vi "Data Processor.vi"() -> (0 "Data Export":T5 {"Data Channels" format="%.2f"})   [LabVIEW 2016]
uses:
  state.ctl
  comm/comm.lvlib
panel:
  in  "LE and RE 2D coils":bool
  in  "Case Constant\n(See Context Help)":bool=TRUE
  in  "3D Convention":T1(ring)=enum."Rotation Vectors"
  in  "Sub Sample Once":bool
  in  "Rex Data File":T2 {"Data -> Additional" format="%.2f"; "Data -> 3D Coil" format="%.2f"}
  in  "Addtional Channels":T3(array[cluster])=[{"Channel No."=0, "Offset Factor"=0.0, "Scaling Factor"=1.0}, {"Channel No."=19, "Offset Factor"=0.0, "Scaling Factor"=1.0}, {"Channel No."=20, "Offset Factor"=0.0, "Scaling Factor"=1.0}, {"Channel No."=21, "Offset Factor"=0.0, "Scaling Factor"=0.1}, {"Channel No."=22, "Offset Factor"=0.0, "Scaling Factor"=0.1}, {"Channel No."=23, "Offset Factor"=0.0, "Scaling Factor"=0.1}, {"Channel No."=24, "Offset Factor"=0.0, "Scaling Factor"=3.05e-05}, {"Channel No."=25, "Offset Factor"=0.0, "Scaling Factor"=3.05e-05}, {"Channel No."=26, "Offset Factor"=0.0, "Scaling Factor"=3.05e-05}, {"Channel No."=27, "Offset Factor"=0.0, "Scaling Factor"=3.05e-05}, {"Channel No."=28, "Offset Factor"=0.0, "Scaling Factor"=1.0}] {"Scaling Factor" format="%.7f"; "Offset Factor" format="%.2f"}
  in  "Coil 0 (Head) : Coil 1 (Left Eye) : Coil 2 (Right Eye)":T4(array[cluster])=[{"Dir and X field channel No."=9, "Dir and Y field channel No."=7, "Dir and Z field channel No."=8, "Tor and X field channel No."=18, "Tor and Y field channel No."=16, "Tor and Z field channel No."=17, "Common Offset Factor"=2048.0, "Common Scaling Factor"=1.0}, {"Dir and X field channel No."=12, "Dir and Y field channel No."=10, "Dir and Z field channel No."=11, "Tor and X field channel No."=15, "Tor and Y field channel No."=13, "Tor and Z field channel No."=14, "Common Offset Factor"=2048.0, "Common Scaling Factor"=1.0}, {"Dir and X field channel No."=3, "Dir and Y field channel No."=1, "Dir and Z field channel No."=2, "Tor and X field channel No."=6, "Tor and Y field channel No."=4, "Tor and Z field channel No."=5, "Common Offset Factor"=2048.0, "Common Scaling Factor"=1.0}] {"Common Scaling Factor" format="%.2f"; "Common Offset Factor" format="%.2f"}
  in  "Export Channel List":u16[](array[ring])=[0, 1, 2, 9, 10, 11, 12, 13, 3, 4, 5, 14, 15, 16, 17, 18, 6, 7, 8, 19, 20, 21, 22, 23, 26, 27, 28, 29, 30, 31, 34, 24, 25, 38] items=["Hz Position-in-Head", "Hy Position-in-Head", "Hx Position-in-Head", "Lz Position-in-Head", "Ly Position-in-Head", "Lx Position-in-Head", "Rz Position-in-Head", "Ry Position-in-Head", "Rx Position-in-Head", "Hx Velocity-in-Head", "Hy Velocity-in-Head", "Hz Velocity-in-Head", "Hl Velocity-in-Head", "Hr Velocity-in-Head", "Lx Velocity-in-Head", "Ly Velocity-in-Head", "Lz Velocity-in-Head", "Ll Velocity-in-Head", "Lr Velocity-in-Head", "Rx Velocity-in-Head", "Ry Velocity-in-Head", "Rz Velocity-in-Head", "Rl Velocity-in-Head", "Rr Velocity-in-Head", "Chair Position", "Chair Velocity", "Button", "Ascension X or ch25", "Ascension X Vel", "Ascension Y", "Ascension Y Vel", "Ascension Z", "Ascension Z Vel", "Ascension q0", "Ascension q1", "Ascension q2", "Ascension q3", "LED", " "]
  out "Processing":bool
  out "All Data":T5 {"Data Channels" format="%.2f"}
  in  "Manually enter the Field Gains":bool
  in  "Selected Calibration File":string
  in  "Calibration File":bool
  in  "Field Gains":i32[][](array[numeric])
  in  "Start Processing":bool
  in  "Channel Plot DY DZ for H LE RE":i32[](array[numeric])=[1, 2, 7, 8, 13, 14, 20]
  in  "Selected Data File":string
  in  "Data File":bool
  in  "Quit":bool
  in  "Stop":bool
  # "Human Data Processor"
  # "AAM 10 april 2002 ver.10"
  # "Coil 2                                   Coil 1                                  Coil 0\n              D                  T                     D                  T                   D                    T"
  # "X"
  # "Y"
  # "Z"
  # "NOTE: EMPTY LIST ALWAYS AT END"
  # "Copyright Americo A. Migliaccio (c) 2002 All Rights Reserved by Author"
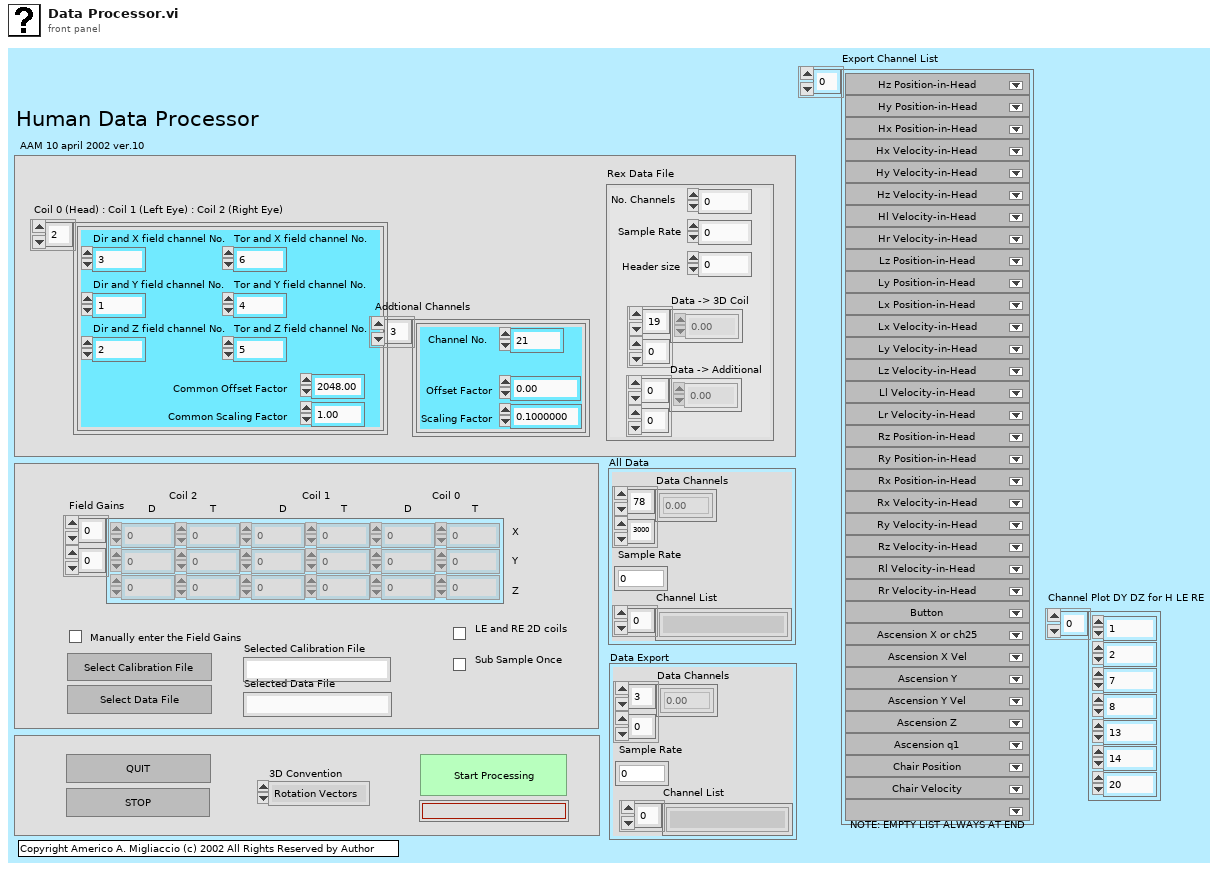
[diagram p1: front panel]
types:
  T1 = enum16{"Rotation Matrix", "Rotation Vectors", "Quaternions", "Fick Angles", "Helmholtz Angles"}
  T2 = cluster{"Header size":i32, "No. Channels":i32, "Sample Rate":i32, "Data -> 3D Coil":dbl[][], "Data -> Additional":dbl[][]}
  T3 = cluster{"Channel No.":i32, "Offset Factor":dbl, "Scaling Factor":dbl}[]
  T4 = cluster{"Dir and X field channel No.":i32, "Dir and Y field channel No.":i32, "Dir and Z field channel No.":i32, "Tor and X field channel No.":i32, "Tor and Y field channel No.":i32, "Tor and Z field channel No.":i32, "Common Offset Factor":dbl, "Common Scaling Factor":dbl}[]
  T5 = cluster{"Data Channels":dbl[][], "Sample Rate":i32, "Channel List":string[]}
  T6 = typedef "state.ctl" = enum16{"Calculate 6 Field/Int Rot Matrix", "SubSample", "Panel Monitoring", "Initialize", "Read 6 Field/Int Calibration File", "Read 6 Field/Int Data File", "Sort 6 Field/Int Channels", "Export Channels", "Stop", "Quit"}
  T7 = enum16{"Position in Space", "Position in Head", "Position in Eye", "Velocity in Space", "Velocity in Head", "Velocity in Eye", "Acceleration in Space", "Acceleration in Head"}
  T8 = cluster{"Coil 0 (Head) : Coil 1 (Left Eye) : Coil 2 (Right Eye)":cluster{"Dir and X field channel No.":i32, "Dir and Y field channel No.":i32, "Dir and Z field channel No.":i32, "Tor and X field channel No.":i32, "Tor and Y field channel No.":i32, "Tor and Z field channel No.":i32, "Common Offset Factor":dbl, "Common Scaling Factor":dbl}[], "Addtional Channels":cluster{"Channel No.":i32, "Offset Factor":dbl, "Scaling Factor":dbl}[], "Selected Calibration File":string, "Selected Data File":string, "Field Gains":i32[][], "Rex Data File":cluster{"Header size":i32, "No. Channels":i32, "Sample Rate":i32, "Data -> 3D Coil":dbl[][], "Data -> Additional":dbl[][]}, "Channel Plot DY DZ for H LE RE":i32[], "All Data":cluster{"Data Channels":dbl[][], "Sample Rate":i32, "Channel List":string[]}}
  T9 = cluster{"Stop ":bool, "Quit":bool, "Calibration File":bool, "Manually enter the Field Gains":bool, "Data File":bool, "Start Processing":bool}
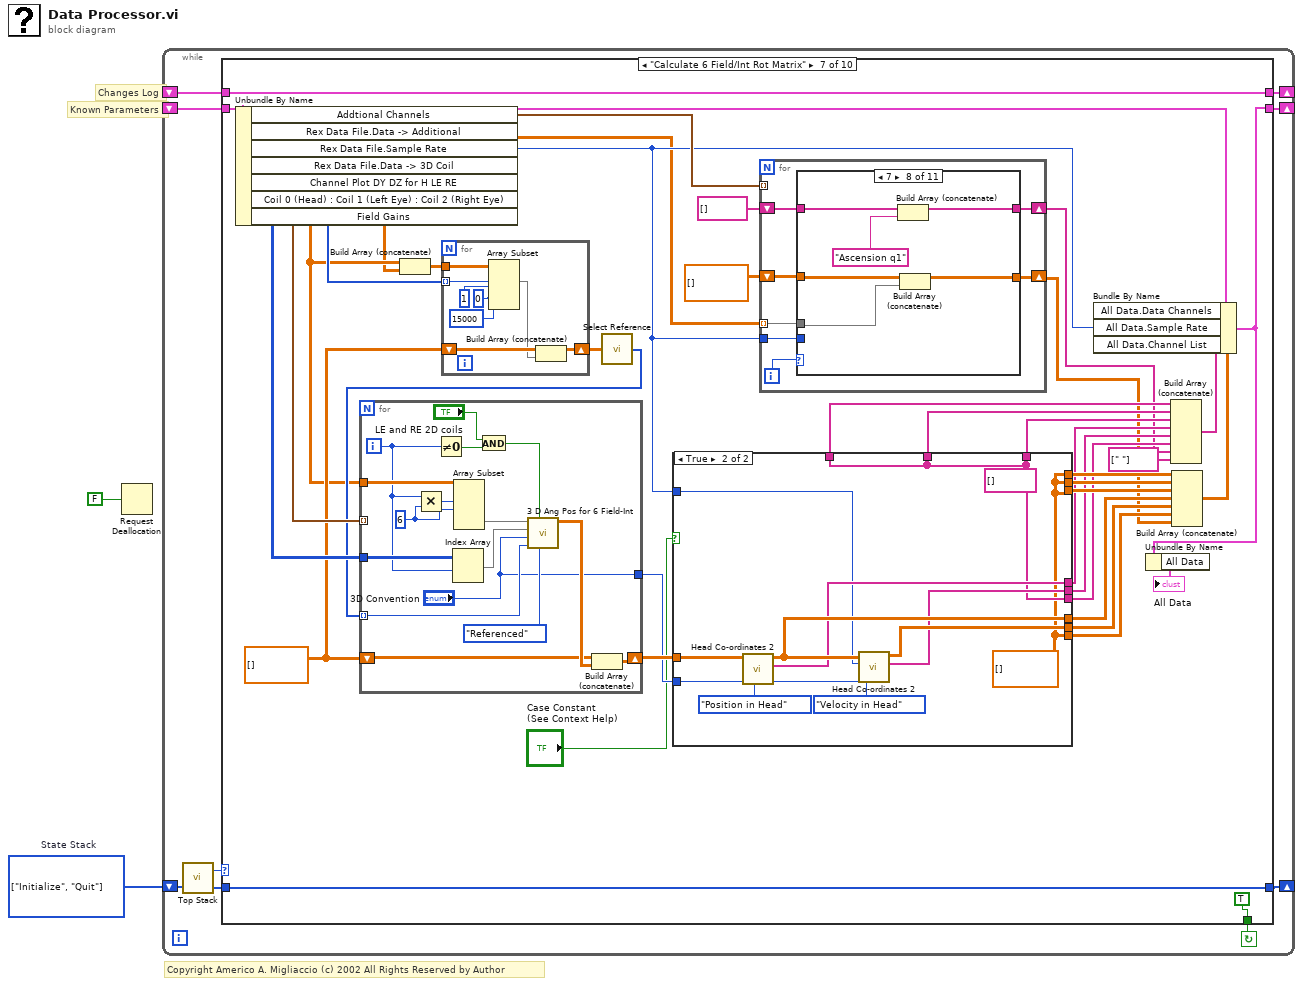
[diagram p0: block diagram]
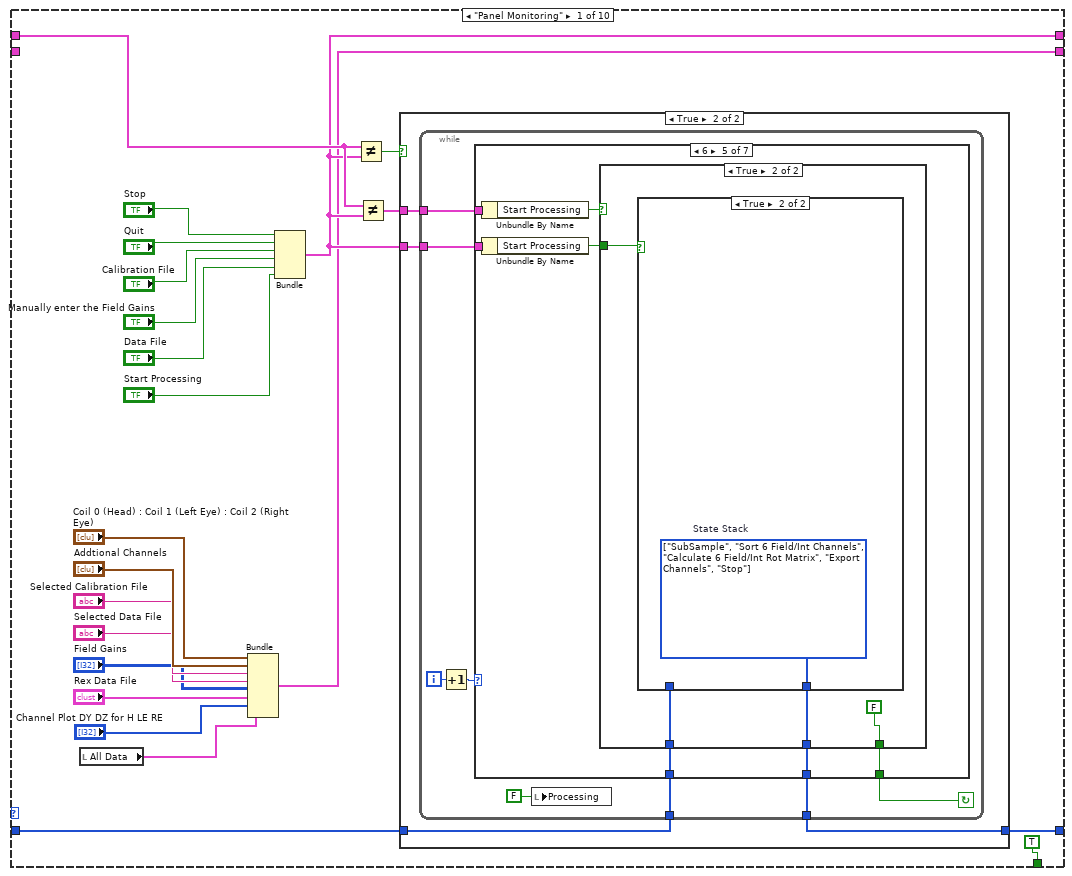
[diagram p2: hidden frame]
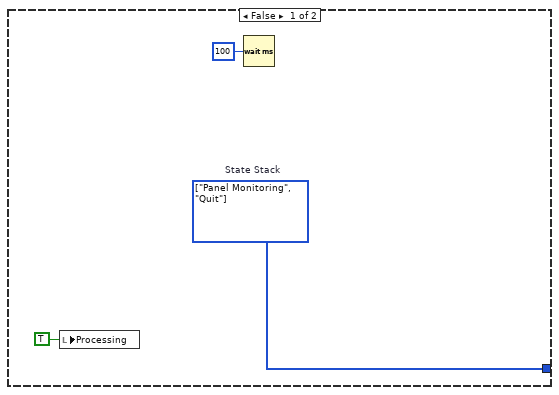
[diagram p3: hidden frame]
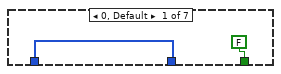
[diagram p4: hidden frame]
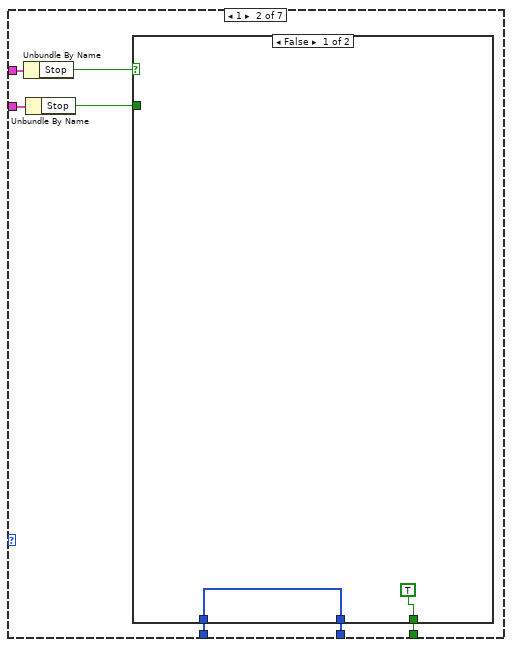
[diagram p5: hidden frame]
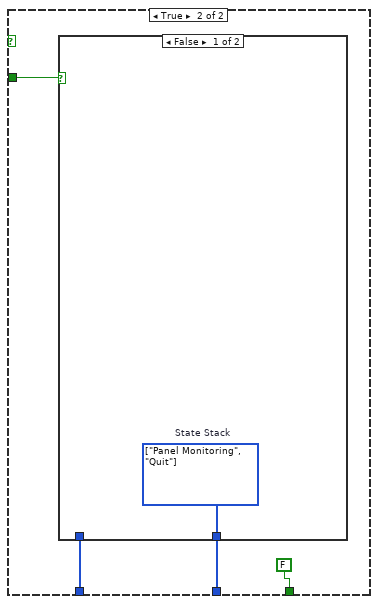
[diagram p6: hidden frame]
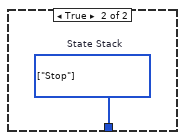
[diagram p7: hidden frame]
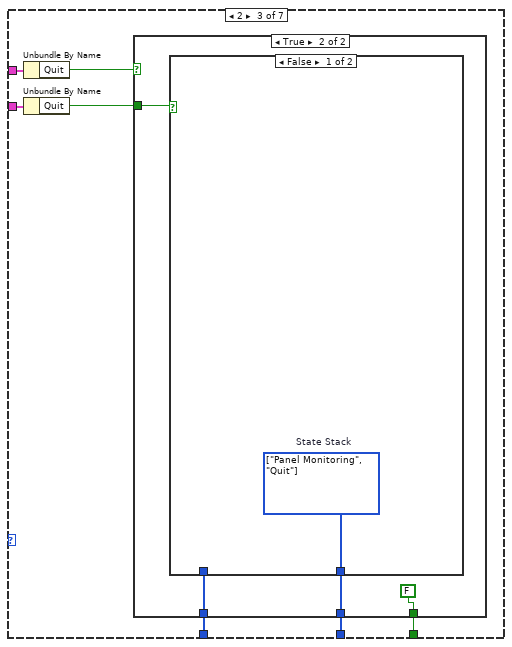
[diagram p8: hidden frame]
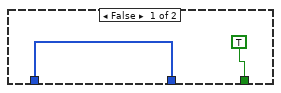
[diagram p9: hidden frame]
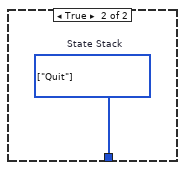
[diagram p10: hidden frame]
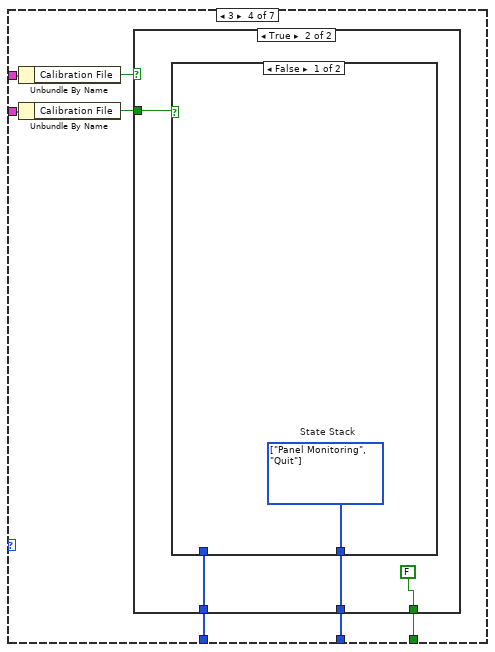
[diagram p11: hidden frame]
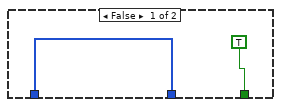
[diagram p12: hidden frame]
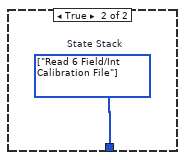
[diagram p13: hidden frame]
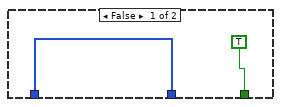
[diagram p14: hidden frame]
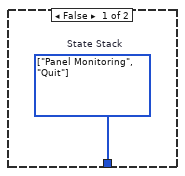
[diagram p15: hidden frame]
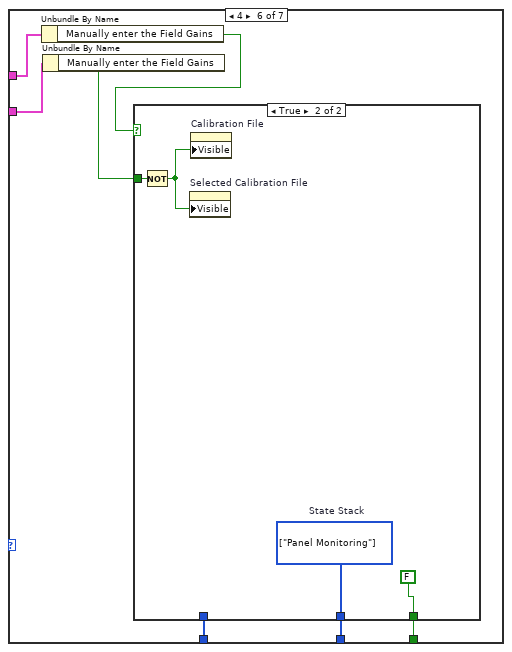
[diagram p16: hidden frame]
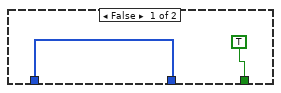
[diagram p17: hidden frame]
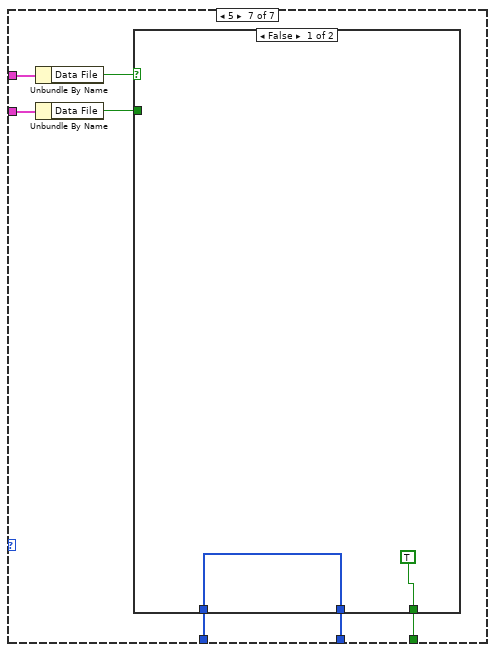
[diagram p18: hidden frame]
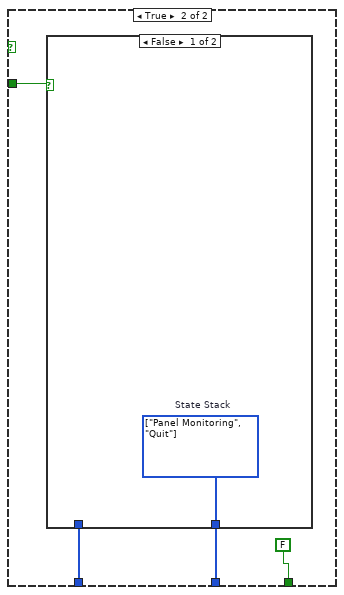
[diagram p19: hidden frame]
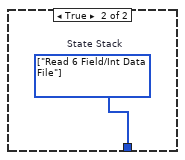
[diagram p20: hidden frame]
diagram:
  w2 = T6[] [enum."Initialize", enum."Quit"] items=["Calculate 6 Field/Int Rot Matrix", "SubSample", "Panel Monitoring", "Initialize", "Read 6 Field/Int Calibration File", "Read 6 Field/Int Data File", "Sort 6 Field/Int Channels", "Export Channels", "Stop", "Quit"]  # State Stack
  # "Copyright Americo A. Migliaccio (c) 2002 All Rights Reserved by Author"
  # "Known Parameters"
  # "Changes Log"
  n1 = Request Deallocation(FALSE ("flag")) -> ()
  n2 = while {
    shift-left: _ -> [w4]
    shift-right: [w3] -> _
    shift-left: _ -> [w6]
    shift-right: [w7] -> _
    shift-left: w2 -> [w11]
    shift-right: [w9] -> _
    stop <- w5 continue-if-true
    n3 = call "Top Stack.vi"("State Stack (in)"=w11) -> ("State Stack (out)"=w10:T6[], "State"=w8:T6)  [unwired: 1 in]
    n4 = case shown="\"Calculate 6 Field/Int Rot Matrix\"" w8 {
      tunnel: w10 -> [w28 _ _ w176 _ w998 w1084 w1237 w1246 w1250]
      tunnel: [w27 w141 w163 w176 w222 w998 w1084 w1237 w1246 w1250] -> w9
      tunnel: [w23 w142 w166 w181 w231 w1003 w1082 w1235 w1244 w1248] -> w7
      tunnel: w6 -> [w30 w142 w166 w181 w231 w1003 w1082 w1235 w1244 w1248]
      tunnel: [TRUE TRUE TRUE TRUE TRUE TRUE TRUE FALSE FALSE FALSE] -> w5
      tunnel: [w17 w140 w165 w178 w230 w997 w1065 w1231 w1243 w1247] -> w3
      tunnel: w4 -> [_ w140 w164 w180 w229 w1000 w1075 w1231 w1243 w1247]
      frame "Panel Monitoring" {
        n5 = local read "All Data"() -> (w12:T5)
        n6 = Bundle("Coil 0 (Head) : Coil 1 (Left Eye) : Coil 2 (Right Eye)"="Coil 0 (Head) : Coil 1 (Left Eye) : Coil 2 (Right Eye)", "Addtional Channels"="Addtional Channels", "Selected Calibration File"="Selected Calibration File", "Selected Data File"="Selected Data File", "Field Gains"="Field Gains", "Rex Data File"="Rex Data File", "Channel Plot DY DZ for H LE RE"="Channel Plot DY DZ for H LE RE", "All Data"=w12) -> (w17:T8)  [unwired: 1 in]
        n7 = Bundle("Stop"="Stop", "Quit"="Quit", "Calibration File"="Calibration File", "Manually enter the Field Gains"="Manually enter the Field Gains", "Data File"="Data File", "Start Processing"="Start Processing") -> (w23:T9)  [unwired: 1 in]
        n8 = Not Equal?(x=w30, y=w23) -> (x != y?=w31:bool)
        n9 = Not Equal?(x=w30, y=w23) -> (x != y?=w29:T9)
        n10 = case shown="True" w31 {
          tunnel: w29 -> [_ w40]
          tunnel: w28 -> [_ w38]
          tunnel: [w36 w39] -> w27
          tunnel: w23 -> [_ w37]
          frame False {
            w36 = T6[] [enum."Panel Monitoring", enum."Quit"] items=["Calculate 6 Field/Int Rot Matrix", "SubSample", "Panel Monitoring", "Initialize", "Read 6 Field/Int Calibration File", "Read 6 Field/Int Data File", "Sort 6 Field/Int Channels", "Export Channels", "Stop", "Quit"]  # State Stack
            n11 = local write "Processing"(TRUE ("Processing")) -> ()
            n12 = Wait (ms)(milliseconds to wait=u32 100) -> ()  [unwired: 1 out]
          }
          frame True {
            n13 = while {
              tunnel: w37 -> [w42]
              tunnel: w38 -> [w45]
              tunnel: [w46] -> w39
              tunnel: w40 -> [w48]
              i -> [w47]
              stop <- w44 continue-if-true
              n14 = Increment(x=w47) -> (x+1=w43:i32)
              n15 = case shown="6" w43 {
                tunnel: w48 -> [_ w57 w72 w87 w102 w117 w130]
                tunnel: [w50 w55 w70 w85 w100 w112 w128] -> w46
                tunnel: w45 -> [w50 w54 w69 w84 w99 w111 w127]
                tunnel: [FALSE w53 w68 w83 w98 w113 w126] -> w44
                tunnel: w42 -> [_ w52 w67 w82 w97 w115 w125]
                frame 0, Default {
                }
                frame 1 {
                  n16 = Unbundle By Name(w57) -> ("Stop"=w56:bool)
                  n17 = Unbundle By Name(w52) -> ("Stop"=w51:bool)
                  n18 = case shown="False" w56 {
                    tunnel: [w59 w63] -> w55
                    tunnel: w54 -> [w59 w61]
                    tunnel: [TRUE FALSE] -> w53
                    tunnel: w51 -> [_ w62]
                    frame False {
                    }
                    frame True {
                      n19 = case shown="False" w62 {
                        tunnel: [w64 w65] -> w63
                        tunnel: w61 -> [_ _]
                        frame False {
                          w64 = T6[] [enum."Panel Monitoring", enum."Quit"] items=["Calculate 6 Field/Int Rot Matrix", "SubSample", "Panel Monitoring", "Initialize", "Read 6 Field/Int Calibration File", "Read 6 Field/Int Data File", "Sort 6 Field/Int Channels", "Export Channels", "Stop", "Quit"]  # State Stack
                        }
                        frame True {
                          w65 = T6[] [enum."Stop"] items=["Calculate 6 Field/Int Rot Matrix", "SubSample", "Panel Monitoring", "Initialize", "Read 6 Field/Int Calibration File", "Read 6 Field/Int Data File", "Sort 6 Field/Int Channels", "Export Channels", "Stop", "Quit"]  # State Stack
                        }
                      }
                    }
                  }
                }
                frame 2 {
                  n20 = Unbundle By Name(w72) -> ("Quit"=w71:bool)
                  n21 = Unbundle By Name(w67) -> ("Quit"=w66:bool)
                  n22 = case shown="True" w71 {
                    tunnel: [w74 w78] -> w70
                    tunnel: w69 -> [w74 w76]
                    tunnel: [TRUE FALSE] -> w68
                    tunnel: w66 -> [_ w77]
                    frame False {
                    }
                    frame True {
                      n23 = case shown="False" w77 {
                        tunnel: [w79 w80] -> w78
                        tunnel: w76 -> [_ _]
                        frame False {
                          w79 = T6[] [enum."Panel Monitoring", enum."Quit"] items=["Calculate 6 Field/Int Rot Matrix", "SubSample", "Panel Monitoring", "Initialize", "Read 6 Field/Int Calibration File", "Read 6 Field/Int Data File", "Sort 6 Field/Int Channels", "Export Channels", "Stop", "Quit"]  # State Stack
                        }
                        frame True {
                          w80 = T6[] [enum."Quit"] items=["Calculate 6 Field/Int Rot Matrix", "SubSample", "Panel Monitoring", "Initialize", "Read 6 Field/Int Calibration File", "Read 6 Field/Int Data File", "Sort 6 Field/Int Channels", "Export Channels", "Stop", "Quit"]  # State Stack
                        }
                      }
                    }
                  }
                }
                frame 3 {
                  n24 = Unbundle By Name(w87) -> ("Calibration File"=w86:bool)
                  n25 = Unbundle By Name(w82) -> ("Calibration File"=w81:bool)
                  n26 = case shown="True" w86 {
                    tunnel: [w89 w93] -> w85
                    tunnel: w84 -> [w89 w92]
                    tunnel: [TRUE FALSE] -> w83
                    tunnel: w81 -> [_ w91]
                    frame False {
                    }
                    frame True {
                      n27 = case shown="False" w91 {
                        tunnel: [w94 w95] -> w93
                        tunnel: w92 -> [_ _]
                        frame False {
                          w94 = T6[] [enum."Panel Monitoring", enum."Quit"] items=["Calculate 6 Field/Int Rot Matrix", "SubSample", "Panel Monitoring", "Initialize", "Read 6 Field/Int Calibration File", "Read 6 Field/Int Data File", "Sort 6 Field/Int Channels", "Export Channels", "Stop", "Quit"]  # State Stack
                        }
                        frame True {
                          w95 = T6[] [enum."Read 6 Field/Int Calibration File"] items=["Calculate 6 Field/Int Rot Matrix", "SubSample", "Panel Monitoring", "Initialize", "Read 6 Field/Int Calibration File", "Read 6 Field/Int Data File", "Sort 6 Field/Int Channels", "Export Channels", "Stop", "Quit"]  # State Stack
                        }
                      }
                    }
                  }
                }
                frame 6 {
                  n28 = Unbundle By Name(w102) -> ("Start Processing"=w101:bool)
                  n29 = Unbundle By Name(w97) -> ("Start Processing"=w96:bool)
                  n30 = case shown="True" w101 {
                    tunnel: [w104 w108] -> w100
                    tunnel: w99 -> [w104 w107]
                    tunnel: [TRUE FALSE] -> w98
                    tunnel: w96 -> [_ w106]
                    frame False {
                    }
                    frame True {
                      n31 = case shown="True" w106 {
                        tunnel: [w109 w110] -> w108
                        tunnel: w107 -> [_ _]
                        frame False {
                          w109 = T6[] [enum."Panel Monitoring", enum."Quit"] items=["Calculate 6 Field/Int Rot Matrix", "SubSample", "Panel Monitoring", "Initialize", "Read 6 Field/Int Calibration File", "Read 6 Field/Int Data File", "Sort 6 Field/Int Channels", "Export Channels", "Stop", "Quit"]  # State Stack
                        }
                        frame True {
                          w110 = T6[] [enum."SubSample", enum."Sort 6 Field/Int Channels", enum."Calculate 6 Field/Int Rot Matrix", enum."Export Channels", enum."Stop"] items=["Calculate 6 Field/Int Rot Matrix", "SubSample", "Panel Monitoring", "Initialize", "Read 6 Field/Int Calibration File", "Read 6 Field/Int Data File", "Sort 6 Field/Int Channels", "Export Channels", "Stop", "Quit"]  # State Stack
                        }
                      }
                    }
                  }
                }
                frame 4 {
                  n32 = Unbundle By Name(w117) -> ("Manually enter the Field Gains"=w116:bool)
                  n33 = Unbundle By Name(w115) -> ("Manually enter the Field Gains"=w114:bool)
                  n34 = case shown="True" w116 {
                    tunnel: w114 -> [_ w123]
                    tunnel: [TRUE FALSE] -> w113
                    tunnel: [w118 w120] -> w112
                    tunnel: w111 -> [w118 _]
                    frame False {
                    }
                    frame True {
                      w120 = T6[] [enum."Panel Monitoring"] items=["Calculate 6 Field/Int Rot Matrix", "SubSample", "Panel Monitoring", "Initialize", "Read 6 Field/Int Calibration File", "Read 6 Field/Int Data File", "Sort 6 Field/Int Channels", "Export Channels", "Stop", "Quit"]  # State Stack
                      n35 = Not(x=w123) -> (.not. x?=w122:bool)
                      n36 = property on="Selected Calibration File" class="Str"("Visible"=w122) -> ()  [unwired: 2 in, 2 out]
                      n37 = property on="Calibration File" class="Bool"("Visible"=w122) -> ()  [unwired: 2 in, 2 out]
                    }
                  }
                }
                frame 5 {
                  n38 = Unbundle By Name(w130) -> ("Data File"=w129:bool)
                  n39 = Unbundle By Name(w125) -> ("Data File"=w124:bool)
                  n40 = case shown="False" w129 {
                    tunnel: [w132 w136] -> w128
                    tunnel: w127 -> [w132 w135]
                    tunnel: [TRUE FALSE] -> w126
                    tunnel: w124 -> [_ w134]
                    frame False {
                    }
                    frame True {
                      n41 = case shown="False" w134 {
                        tunnel: [w137 w138] -> w136
                        tunnel: w135 -> [_ _]
                        frame False {
                          w137 = T6[] [enum."Panel Monitoring", enum."Quit"] items=["Calculate 6 Field/Int Rot Matrix", "SubSample", "Panel Monitoring", "Initialize", "Read 6 Field/Int Calibration File", "Read 6 Field/Int Data File", "Sort 6 Field/Int Channels", "Export Channels", "Stop", "Quit"]  # State Stack
                        }
                        frame True {
                          w138 = T6[] [enum."Read 6 Field/Int Data File"] items=["Calculate 6 Field/Int Rot Matrix", "SubSample", "Panel Monitoring", "Initialize", "Read 6 Field/Int Calibration File", "Read 6 Field/Int Data File", "Sort 6 Field/Int Channels", "Export Channels", "Stop", "Quit"]  # State Stack
                        }
                      }
                    }
                  }
                }
              }
              n42 = local write "Processing"(FALSE ("Processing")) -> ()
            }
          }
        }
      }
      frame "Initialize" {
        w141 = T6[] [enum."Panel Monitoring", enum."Quit"] items=["Calculate 6 Field/Int Rot Matrix", "SubSample", "Panel Monitoring", "Initialize", "Read 6 Field/Int Calibration File", "Read 6 Field/Int Data File", "Sort 6 Field/Int Channels", "Export Channels", "Stop", "Quit"]  # State Stack
        "Processing" <- FALSE ("Processing")
      }
      frame "Read 6 Field/Int Calibration File" {
        w153 = 6 ("Array Length")
        w156 = "/" ("Substring")
        w163 = T6[] [enum."Panel Monitoring"] items=["Calculate 6 Field/Int Rot Matrix", "SubSample", "Panel Monitoring", "Initialize", "Read 6 Field/Int Calibration File", "Read 6 Field/Int Data File", "Sort 6 Field/Int Channels", "Export Channels", "Stop", "Quit"]  # State Stack
        n43 = File Dialog(7:"Select Field Gains File" ("prompt")) -> (0:w144:errorcluster, 3:w159:path)  [unwired: 6 in, 2 out]
        n44 = Unbundle(w144) -> ()  [unwired: 3 out]
        n45 = call <vilib>:"Read Characters From File.vi"("file path (dialog if empty)"=w159) -> ("character string"=w160:string)  [unwired: 5 in, 3 out]
        n46 = Strip Path(path=w159) -> (stripped path=w158:path, name=w155:string)
        n47 = Strip Path(path=w158) -> (name=w157:string)  [unwired: 1 out]
        n48 = while {
          shift-left: u32 0 -> [w171]
          shift-right: [w172] -> _
          tunnel: w160 -> [w173]
          tunnel: [w174] -> w152 mode=indexing
          stop <- w168 continue-if-true
          n49 = Scan From String(format string="%5d" ("Format String"), input string=w173, initial scan location=w171) -> (offset past scan=w172:u32, error out=w170:errorcluster, output 1=w174:i32)  [unwired: 2 in, 1 out]
          n50 = Unbundle By Name(w170) -> ("status"=w169:bool)
          n51 = Not(x=w169) -> (.not. x?=w168:bool)
        }
        n52 = Concatenate Strings(w156, w157, w156, w155) -> (w145:string)
        n53 = local write "Selected Calibration File"(w145) -> ()
        n54 = Array Subset(array=w152, index=0 ("Array Index"), length=w153) -> (w149:i32[])
        n55 = Array Subset(array=w152, index=6 ("Array Index"), length=w153) -> (w148:i32[])
        n56 = Array Subset(array=w152, index=12 ("Array Index"), length=w153) -> (w147:i32[])
        n57 = Build Array(w149, w148, w147) -> (w146:i32[][])
        n58 = Bundle By Name(cluster=w164, "Selected Calibration File"=w145, "Field Gains"=w146) -> (w165:T8)
        n59 = local write "Field Gains"(w146) -> ()
      }
      frame "SubSample" {
        n60 = case shown="True" "Sub Sample Once" {
          tunnel: w180 -> [w183 w190]
          tunnel: [w183 w184] -> w178
          frame False {
          }
          frame True {
            n61 = Unbundle By Name(w190) -> ("Rex Data File.Data -> 3D Coil"=w186:dbl[][], "Rex Data File.Sample Rate"=w189:i32)
            n62 = Quotient & Remainder(x=w189, y=2) -> (floor(x/y)=w187:i32)  [unwired: 1 out]
            n63 = for {
              tunnel: w186 -> [w192] mode=indexing
              tunnel: [w191] -> w185 mode=indexing
              n64 = Decimate 1D Array(w192) -> (w191:dbl[])  [unwired: 1 out]
            }
            n65 = Bundle By Name(cluster=w190, "Rex Data File.Data -> 3D Coil"=w185, "Rex Data File.Sample Rate"=w187) -> (w184:T8)
          }
        }
        n66 = Unbundle By Name(w178) -> ("Rex Data File"=w177:T2)
        n67 = local write "Rex Data File"(w177) -> ()
      }
      frame "Read 6 Field/Int Data File" {
        w216 = "msecstp" ("search string/char (-)")
        w217 = "achan" ("search string/char (-)")
        w225 = "/" ("Substring")
        w222 = T6[] [enum."Panel Monitoring"] items=["Calculate 6 Field/Int Rot Matrix", "SubSample", "Panel Monitoring", "Initialize", "Read 6 Field/Int Calibration File", "Read 6 Field/Int Data File", "Sort 6 Field/Int Channels", "Export Channels", "Stop", "Quit"]  # State Stack
        n68 = File Dialog(7:"Select Field Data File" ("prompt")) -> (0:w193:errorcluster, 3:w196:path)  [unwired: 6 in, 2 out]
        n69 = Unbundle(w193) -> ()  [unwired: 3 out]
        n70 = call <vilib>:"Read Characters From File.vi"("file path (dialog if empty)"=w196, "number of characters (all:-1)"=1000) -> ("character string"=w208:string)  [unwired: 4 in, 3 out]
        n71 = Strip Path(path=w196) -> (stripped path=w227:path, name=w224:string)
        n72 = Strip Path(path=w227) -> (name=w226:string)  [unwired: 1 out]
        n73 = Search/Split String(string=w208, search string/char (-)="\u0000") -> (substring before match=w211:string)  [unwired: 1 in, 2 out]
        n74 = Concatenate Strings(w225, w226, w225, w224) -> (w201:string)
        n75 = local write "Selected Data File"(w201) -> ()
        n76 = String Length(string=w211) -> (length=w206:i32)
        n77 = Add(x=1, y=w206) -> (x+y=w203:i32)
        n78 = call <vilib>:"Read From I16 File.vi"("start of read offset (bytes:0)"=w203, "file path (dialog if empty)"=w196) -> ("1D array"=w194:i16[])  [unwired: 5 in, 4 out]
        n79 = Search/Split String(string=w211, search string/char (-)=w217) -> (offset of match=w220:i32)  [unwired: 1 in, 2 out]
        n80 = Search/Split String(string=w211, search string/char (-)=w216) -> (offset of match=w213:i32)  [unwired: 1 in, 2 out]
        n81 = String Length(string=w217) -> (length=w218:i32)
        n82 = String Length(string=w216) -> (length=w215:i32)
        n83 = Swap Bytes(anything=w194) -> (byte swapped=w195:i16[])
        n84 = Add(x=w220, y=w218) -> (x+y=w219:i32)
        n85 = Add(x=w213, y=w215) -> (x+y=w214:i32)
        n86 = Scan From String(format string="%d" ("regular expression"), input string=w211, initial scan location=w219) -> (output 1=w198:i32)  [unwired: 2 in, 3 out]
        n87 = Scan From String(format string="%d" ("regular expression"), input string=w211, initial scan location=w214) -> (output 1=w209:i32)  [unwired: 2 in, 3 out]
        n88 = To Double Precision Float(number=w195) -> (double precision float=w199:dbl[])
        n89 = Quotient & Remainder(x=1000, y=w209) -> (floor(x/y)=w204:i32)  [unwired: 1 out]
        n90 = case shown="18" w198 {
          tunnel: w199 -> [w252 w273 w295 w318 w342 w367 w393 w420 w448 w477 w507 w538 w570 w603 w637 w672 w708 w745 w783 w822 w862 w903 w945 w988]
          tunnel: [w233 w254 w276 w299 w323 w348 w374 w401 w429 w458 w488 w519 w551 w584 w618 w653 w689 w726 w764 w803 w843 w884 w926 w969] -> w197
          frame 18 {
            n91 = Decimate 1D Array(w252) -> (w251:dbl[], w250:dbl[], w249:dbl[], w248:dbl[], w247:dbl[], w246:dbl[], w245:dbl[], w244:dbl[], w243:dbl[], w242:dbl[], w241:dbl[], w240:dbl[], w239:dbl[], w238:dbl[], w237:dbl[], w236:dbl[], w235:dbl[], w234:dbl[])
            n92 = Build Array(w251, w250, w249, w248, w247, w246, w245, w244, w243, w242, w241, w240, w239, w238, w237, w236, w235, w234) -> (w233:dbl[][])
          }
          frame 19 {
            n93 = Decimate 1D Array(w273) -> (w272:dbl[], w271:dbl[], w270:dbl[], w269:dbl[], w268:dbl[], w267:dbl[], w266:dbl[], w265:dbl[], w264:dbl[], w263:dbl[], w262:dbl[], w261:dbl[], w260:dbl[], w259:dbl[], w258:dbl[], w257:dbl[], w256:dbl[], w255:dbl[], w253:dbl[])
            n94 = Build Array(w272, w271, w270, w269, w268, w267, w266, w265, w264, w263, w262, w261, w260, w259, w258, w257, w256, w255, w253) -> (w254:dbl[][])
          }
          frame 20 {
            n95 = Decimate 1D Array(w295) -> (w294:dbl[], w293:dbl[], w292:dbl[], w291:dbl[], w290:dbl[], w289:dbl[], w288:dbl[], w287:dbl[], w286:dbl[], w285:dbl[], w284:dbl[], w283:dbl[], w282:dbl[], w281:dbl[], w280:dbl[], w279:dbl[], w278:dbl[], w277:dbl[], w275:dbl[], w274:dbl[])
            n96 = Build Array(w294, w293, w292, w291, w290, w289, w288, w287, w286, w285, w284, w283, w282, w281, w280, w279, w278, w277, w275, w274) -> (w276:dbl[][])
          }
          frame 21, Default {
            n97 = Decimate 1D Array(w318) -> (w317:dbl[], w316:dbl[], w315:dbl[], w314:dbl[], w313:dbl[], w312:dbl[], w311:dbl[], w310:dbl[], w309:dbl[], w308:dbl[], w307:dbl[], w306:dbl[], w305:dbl[], w304:dbl[], w303:dbl[], w302:dbl[], w301:dbl[], w300:dbl[], w298:dbl[], w297:dbl[], w296:dbl[])
            n98 = Build Array(w317, w316, w315, w314, w313, w312, w311, w310, w309, w308, w307, w306, w305, w304, w303, w302, w301, w300, w298, w297, w296) -> (w299:dbl[][])
          }
          frame 22 {
            n99 = Decimate 1D Array(w342) -> (w341:dbl[], w340:dbl[], w339:dbl[], w338:dbl[], w337:dbl[], w336:dbl[], w335:dbl[], w334:dbl[], w333:dbl[], w332:dbl[], w331:dbl[], w330:dbl[], w329:dbl[], w328:dbl[], w327:dbl[], w326:dbl[], w325:dbl[], w324:dbl[], w322:dbl[], w321:dbl[], w320:dbl[], w319:dbl[])
            n100 = Build Array(w341, w340, w339, w338, w337, w336, w335, w334, w333, w332, w331, w330, w329, w328, w327, w326, w325, w324, w322, w321, w320, w319) -> (w323:dbl[][])
          }
          frame 23 {
            n101 = Decimate 1D Array(w367) -> (w366:dbl[], w365:dbl[], w364:dbl[], w363:dbl[], w362:dbl[], w361:dbl[], w360:dbl[], w359:dbl[], w358:dbl[], w357:dbl[], w356:dbl[], w355:dbl[], w354:dbl[], w353:dbl[], w352:dbl[], w351:dbl[], w350:dbl[], w349:dbl[], w347:dbl[], w346:dbl[], w345:dbl[], w344:dbl[], w343:dbl[])
            n102 = Build Array(w366, w365, w364, w363, w362, w361, w360, w359, w358, w357, w356, w355, w354, w353, w352, w351, w350, w349, w347, w346, w345, w344, w343) -> (w348:dbl[][])
          }
          frame 24 {
            n103 = Decimate 1D Array(w393) -> (w392:dbl[], w391:dbl[], w390:dbl[], w389:dbl[], w388:dbl[], w387:dbl[], w386:dbl[], w385:dbl[], w384:dbl[], w383:dbl[], w382:dbl[], w381:dbl[], w380:dbl[], w379:dbl[], w378:dbl[], w377:dbl[], w376:dbl[], w375:dbl[], w373:dbl[], w372:dbl[], w371:dbl[], w370:dbl[], w369:dbl[], w368:dbl[])
            n104 = Build Array(w392, w391, w390, w389, w388, w387, w386, w385, w384, w383, w382, w381, w380, w379, w378, w377, w376, w375, w373, w372, w371, w370, w369, w368) -> (w374:dbl[][])
          }
          frame 25 {
            n105 = Decimate 1D Array(w420) -> (w419:dbl[], w418:dbl[], w417:dbl[], w416:dbl[], w415:dbl[], w414:dbl[], w413:dbl[], w412:dbl[], w411:dbl[], w410:dbl[], w409:dbl[], w408:dbl[], w407:dbl[], w406:dbl[], w405:dbl[], w404:dbl[], w403:dbl[], w402:dbl[], w400:dbl[], w399:dbl[], w398:dbl[], w397:dbl[], w396:dbl[], w395:dbl[], w394:dbl[])
            n106 = Build Array(w419, w418, w417, w416, w415, w414, w413, w412, w411, w410, w409, w408, w407, w406, w405, w404, w403, w402, w400, w399, w398, w397, w396, w395, w394) -> (w401:dbl[][])
          }
          frame 26 {
            n107 = Decimate 1D Array(w448) -> (w447:dbl[], w446:dbl[], w445:dbl[], w444:dbl[], w443:dbl[], w442:dbl[], w441:dbl[], w440:dbl[], w439:dbl[], w438:dbl[], w437:dbl[], w436:dbl[], w435:dbl[], w434:dbl[], w433:dbl[], w432:dbl[], w431:dbl[], w430:dbl[], w428:dbl[], w427:dbl[], w426:dbl[], w425:dbl[], w424:dbl[], w423:dbl[], w422:dbl[], w421:dbl[])
            n108 = Build Array(w447, w446, w445, w444, w443, w442, w441, w440, w439, w438, w437, w436, w435, w434, w433, w432, w431, w430, w428, w427, w426, w425, w424, w423, w422, w421) -> (w429:dbl[][])
          }
          frame 27 {
            n109 = Decimate 1D Array(w477) -> (w476:dbl[], w475:dbl[], w474:dbl[], w473:dbl[], w472:dbl[], w471:dbl[], w470:dbl[], w469:dbl[], w468:dbl[], w467:dbl[], w466:dbl[], w465:dbl[], w464:dbl[], w463:dbl[], w462:dbl[], w461:dbl[], w460:dbl[], w459:dbl[], w457:dbl[], w456:dbl[], w455:dbl[], w454:dbl[], w453:dbl[], w452:dbl[], w451:dbl[], w449:dbl[], w450:dbl[])
            n110 = Build Array(w476, w475, w474, w473, w472, w471, w470, w469, w468, w467, w466, w465, w464, w463, w462, w461, w460, w459, w457, w456, w455, w454, w453, w452, w451, w449, w450) -> (w458:dbl[][])
          }
          frame 28 {
            n111 = Decimate 1D Array(w507) -> (w506:dbl[], w505:dbl[], w504:dbl[], w503:dbl[], w502:dbl[], w501:dbl[], w500:dbl[], w499:dbl[], w498:dbl[], w497:dbl[], w496:dbl[], w495:dbl[], w494:dbl[], w493:dbl[], w492:dbl[], w491:dbl[], w490:dbl[], w489:dbl[], w487:dbl[], w486:dbl[], w485:dbl[], w484:dbl[], w483:dbl[], w482:dbl[], w481:dbl[], w480:dbl[], w479:dbl[], w478:dbl[])
            n112 = Build Array(w506, w505, w504, w503, w502, w501, w500, w499, w498, w497, w496, w495, w494, w493, w492, w491, w490, w489, w487, w486, w485, w484, w483, w482, w481, w480, w479, w478) -> (w488:dbl[][])
          }
          frame 29 {
            n113 = Decimate 1D Array(w538) -> (w537:dbl[], w536:dbl[], w535:dbl[], w534:dbl[], w533:dbl[], w532:dbl[], w531:dbl[], w530:dbl[], w529:dbl[], w528:dbl[], w527:dbl[], w526:dbl[], w525:dbl[], w524:dbl[], w523:dbl[], w522:dbl[], w521:dbl[], w520:dbl[], w518:dbl[], w517:dbl[], w516:dbl[], w515:dbl[], w514:dbl[], w513:dbl[], w512:dbl[], w511:dbl[], w510:dbl[], w509:dbl[], w508:dbl[])
            n114 = Build Array(w537, w536, w535, w534, w533, w532, w531, w530, w529, w528, w527, w526, w525, w524, w523, w522, w521, w520, w518, w517, w516, w515, w514, w513, w512, w511, w510, w509, w508) -> (w519:dbl[][])
          }
          frame 30 {
            n115 = Decimate 1D Array(w570) -> (w569:dbl[], w568:dbl[], w567:dbl[], w566:dbl[], w565:dbl[], w564:dbl[], w563:dbl[], w562:dbl[], w561:dbl[], w560:dbl[], w559:dbl[], w558:dbl[], w557:dbl[], w556:dbl[], w555:dbl[], w554:dbl[], w553:dbl[], w552:dbl[], w550:dbl[], w549:dbl[], w548:dbl[], w547:dbl[], w546:dbl[], w545:dbl[], w544:dbl[], w543:dbl[], w542:dbl[], w541:dbl[], w540:dbl[], w539:dbl[])
            n116 = Build Array(w569, w568, w567, w566, w565, w564, w563, w562, w561, w560, w559, w558, w557, w556, w555, w554, w553, w552, w550, w549, w548, w547, w546, w545, w544, w543, w542, w541, w540, w539) -> (w551:dbl[][])
          }
          frame 31 {
            n117 = Decimate 1D Array(w603) -> (w602:dbl[], w601:dbl[], w600:dbl[], w599:dbl[], w598:dbl[], w597:dbl[], w596:dbl[], w595:dbl[], w594:dbl[], w593:dbl[], w592:dbl[], w591:dbl[], w590:dbl[], w589:dbl[], w588:dbl[], w587:dbl[], w586:dbl[], w585:dbl[], w583:dbl[], w582:dbl[], w581:dbl[], w580:dbl[], w579:dbl[], w578:dbl[], w577:dbl[], w576:dbl[], w575:dbl[], w574:dbl[], w573:dbl[], w572:dbl[], w571:dbl[])
            n118 = Build Array(w602, w601, w600, w599, w598, w597, w596, w595, w594, w593, w592, w591, w590, w589, w588, w587, w586, w585, w583, w582, w581, w580, w579, w578, w577, w576, w575, w574, w573, w572, w571) -> (w584:dbl[][])
          }
          frame 32 {
            n119 = Decimate 1D Array(w637) -> (w636:dbl[], w635:dbl[], w634:dbl[], w633:dbl[], w632:dbl[], w631:dbl[], w630:dbl[], w629:dbl[], w628:dbl[], w627:dbl[], w626:dbl[], w625:dbl[], w624:dbl[], w623:dbl[], w622:dbl[], w621:dbl[], w620:dbl[], w619:dbl[], w617:dbl[], w616:dbl[], w615:dbl[], w614:dbl[], w613:dbl[], w612:dbl[], w611:dbl[], w610:dbl[], w609:dbl[], w608:dbl[], w607:dbl[], w606:dbl[], w605:dbl[], w604:dbl[])
            n120 = Build Array(w636, w635, w634, w633, w632, w631, w630, w629, w628, w627, w626, w625, w624, w623, w622, w621, w620, w619, w617, w616, w615, w614, w613, w612, w611, w610, w609, w608, w607, w606, w605, w604) -> (w618:dbl[][])
          }
          frame 33 {
            n121 = Decimate 1D Array(w672) -> (w671:dbl[], w670:dbl[], w669:dbl[], w668:dbl[], w667:dbl[], w666:dbl[], w665:dbl[], w664:dbl[], w663:dbl[], w662:dbl[], w661:dbl[], w660:dbl[], w659:dbl[], w658:dbl[], w657:dbl[], w656:dbl[], w655:dbl[], w654:dbl[], w652:dbl[], w651:dbl[], w650:dbl[], w649:dbl[], w648:dbl[], w647:dbl[], w646:dbl[], w645:dbl[], w644:dbl[], w643:dbl[], w642:dbl[], w641:dbl[], w640:dbl[], w639:dbl[], w638:dbl[])
            n122 = Build Array(w671, w670, w669, w668, w667, w666, w665, w664, w663, w662, w661, w660, w659, w658, w657, w656, w655, w654, w652, w651, w650, w649, w648, w647, w646, w645, w644, w643, w642, w641, w640, w639, w638) -> (w653:dbl[][])
          }
          frame 34 {
            n123 = Decimate 1D Array(w708) -> (w707:dbl[], w706:dbl[], w705:dbl[], w704:dbl[], w703:dbl[], w702:dbl[], w701:dbl[], w700:dbl[], w699:dbl[], w698:dbl[], w697:dbl[], w696:dbl[], w695:dbl[], w694:dbl[], w693:dbl[], w692:dbl[], w691:dbl[], w690:dbl[], w688:dbl[], w687:dbl[], w686:dbl[], w685:dbl[], w684:dbl[], w683:dbl[], w682:dbl[], w681:dbl[], w680:dbl[], w679:dbl[], w678:dbl[], w677:dbl[], w676:dbl[], w675:dbl[], w674:dbl[], w673:dbl[])
            n124 = Build Array(w707, w706, w705, w704, w703, w702, w701, w700, w699, w698, w697, w696, w695, w694, w693, w692, w691, w690, w688, w687, w686, w685, w684, w683, w682, w681, w680, w679, w678, w677, w676, w675, w674, w673) -> (w689:dbl[][])
          }
          frame 35 {
            n125 = Decimate 1D Array(w745) -> (w744:dbl[], w743:dbl[], w742:dbl[], w741:dbl[], w740:dbl[], w739:dbl[], w738:dbl[], w737:dbl[], w736:dbl[], w735:dbl[], w734:dbl[], w733:dbl[], w732:dbl[], w731:dbl[], w730:dbl[], w729:dbl[], w728:dbl[], w727:dbl[], w725:dbl[], w724:dbl[], w723:dbl[], w722:dbl[], w721:dbl[], w720:dbl[], w719:dbl[], w718:dbl[], w717:dbl[], w716:dbl[], w715:dbl[], w714:dbl[], w713:dbl[], w712:dbl[], w711:dbl[], w710:dbl[], w709:dbl[])
            n126 = Build Array(w744, w743, w742, w741, w740, w739, w738, w737, w736, w735, w734, w733, w732, w731, w730, w729, w728, w727, w725, w724, w723, w722, w721, w720, w719, w718, w717, w716, w715, w714, w713, w712, w711, w710, w709) -> (w726:dbl[][])
          }
          frame 36 {
            n127 = Decimate 1D Array(w783) -> (w782:dbl[], w781:dbl[], w780:dbl[], w779:dbl[], w778:dbl[], w777:dbl[], w776:dbl[], w775:dbl[], w774:dbl[], w773:dbl[], w772:dbl[], w771:dbl[], w770:dbl[], w769:dbl[], w768:dbl[], w767:dbl[], w766:dbl[], w765:dbl[], w763:dbl[], w762:dbl[], w761:dbl[], w760:dbl[], w759:dbl[], w758:dbl[], w757:dbl[], w756:dbl[], w755:dbl[], w754:dbl[], w753:dbl[], w752:dbl[], w751:dbl[], w750:dbl[], w749:dbl[], w748:dbl[], w747:dbl[], w746:dbl[])
            n128 = Build Array(w782, w781, w780, w779, w778, w777, w776, w775, w774, w773, w772, w771, w770, w769, w768, w767, w766, w765, w763, w762, w761, w760, w759, w758, w757, w756, w755, w754, w753, w752, w751, w750, w749, w748, w747, w746) -> (w764:dbl[][])
          }
          frame 37 {
            n129 = Decimate 1D Array(w822) -> (w821:dbl[], w820:dbl[], w819:dbl[], w818:dbl[], w817:dbl[], w816:dbl[], w815:dbl[], w814:dbl[], w813:dbl[], w812:dbl[], w811:dbl[], w810:dbl[], w809:dbl[], w808:dbl[], w807:dbl[], w806:dbl[], w805:dbl[], w804:dbl[], w802:dbl[], w801:dbl[], w800:dbl[], w799:dbl[], w798:dbl[], w797:dbl[], w796:dbl[], w795:dbl[], w794:dbl[], w793:dbl[], w792:dbl[], w791:dbl[], w790:dbl[], w789:dbl[], w788:dbl[], w787:dbl[], w786:dbl[], w784:dbl[], w785:dbl[])
            n130 = Build Array(w821, w820, w819, w818, w817, w816, w815, w814, w813, w812, w811, w810, w809, w808, w807, w806, w805, w804, w802, w801, w800, w799, w798, w797, w796, w795, w794, w793, w792, w791, w790, w789, w788, w787, w786, w784, w785) -> (w803:dbl[][])
          }
          frame 38 {
            n131 = Decimate 1D Array(w862) -> (w861:dbl[], w860:dbl[], w859:dbl[], w858:dbl[], w857:dbl[], w856:dbl[], w855:dbl[], w854:dbl[], w853:dbl[], w852:dbl[], w851:dbl[], w850:dbl[], w849:dbl[], w848:dbl[], w847:dbl[], w846:dbl[], w845:dbl[], w844:dbl[], w842:dbl[], w841:dbl[], w840:dbl[], w839:dbl[], w838:dbl[], w837:dbl[], w836:dbl[], w835:dbl[], w834:dbl[], w833:dbl[], w832:dbl[], w831:dbl[], w830:dbl[], w829:dbl[], w828:dbl[], w827:dbl[], w826:dbl[], w823:dbl[], w824:dbl[], w825:dbl[])
            n132 = Build Array(w861, w860, w859, w858, w857, w856, w855, w854, w853, w852, w851, w850, w849, w848, w847, w846, w845, w844, w842, w841, w840, w839, w838, w837, w836, w835, w834, w833, w832, w831, w830, w829, w828, w827, w826, w823, w824, w825) -> (w843:dbl[][])
          }
          frame 39 {
            n133 = Decimate 1D Array(w903) -> (w902:dbl[], w901:dbl[], w900:dbl[], w899:dbl[], w898:dbl[], w897:dbl[], w896:dbl[], w895:dbl[], w894:dbl[], w893:dbl[], w892:dbl[], w891:dbl[], w890:dbl[], w889:dbl[], w888:dbl[], w887:dbl[], w886:dbl[], w885:dbl[], w883:dbl[], w882:dbl[], w881:dbl[], w880:dbl[], w879:dbl[], w878:dbl[], w877:dbl[], w876:dbl[], w875:dbl[], w874:dbl[], w873:dbl[], w872:dbl[], w871:dbl[], w870:dbl[], w869:dbl[], w868:dbl[], w867:dbl[], w863:dbl[], w864:dbl[], w865:dbl[], w866:dbl[])
            n134 = Build Array(w902, w901, w900, w899, w898, w897, w896, w895, w894, w893, w892, w891, w890, w889, w888, w887, w886, w885, w883, w882, w881, w880, w879, w878, w877, w876, w875, w874, w873, w872, w871, w870, w869, w868, w867, w863, w864, w865, w866) -> (w884:dbl[][])
          }
          frame 40 {
            n135 = Decimate 1D Array(w945) -> (w944:dbl[], w943:dbl[], w942:dbl[], w941:dbl[], w940:dbl[], w939:dbl[], w938:dbl[], w937:dbl[], w936:dbl[], w935:dbl[], w934:dbl[], w933:dbl[], w932:dbl[], w931:dbl[], w930:dbl[], w929:dbl[], w928:dbl[], w927:dbl[], w925:dbl[], w924:dbl[], w923:dbl[], w922:dbl[], w921:dbl[], w920:dbl[], w919:dbl[], w918:dbl[], w917:dbl[], w916:dbl[], w915:dbl[], w914:dbl[], w913:dbl[], w912:dbl[], w911:dbl[], w910:dbl[], w909:dbl[], w904:dbl[], w905:dbl[], w906:dbl[], w907:dbl[], w908:dbl[])
            n136 = Build Array(w944, w943, w942, w941, w940, w939, w938, w937, w936, w935, w934, w933, w932, w931, w930, w929, w928, w927, w925, w924, w923, w922, w921, w920, w919, w918, w917, w916, w915, w914, w913, w912, w911, w910, w909, w904, w905, w906, w907, w908) -> (w926:dbl[][])
          }
          frame 41 {
            n137 = Decimate 1D Array(w988) -> (w987:dbl[], w986:dbl[], w985:dbl[], w984:dbl[], w983:dbl[], w982:dbl[], w981:dbl[], w980:dbl[], w979:dbl[], w978:dbl[], w977:dbl[], w976:dbl[], w975:dbl[], w974:dbl[], w973:dbl[], w972:dbl[], w971:dbl[], w970:dbl[], w968:dbl[], w967:dbl[], w966:dbl[], w965:dbl[], w964:dbl[], w963:dbl[], w962:dbl[], w961:dbl[], w960:dbl[], w959:dbl[], w958:dbl[], w957:dbl[], w956:dbl[], w955:dbl[], w954:dbl[], w953:dbl[], w952:dbl[], w946:dbl[], w947:dbl[], w948:dbl[], w949:dbl[], w950:dbl[], w951:dbl[])
            n138 = Build Array(w987, w986, w985, w984, w983, w982, w981, w980, w979, w978, w977, w976, w975, w974, w973, w972, w971, w970, w968, w967, w966, w965, w964, w963, w962, w961, w960, w959, w958, w957, w956, w955, w954, w953, w952, w946, w947, w948, w949, w950, w951) -> (w969:dbl[][])
          }
        }
        n139 = local read "Rex Data File"() -> (w202:T2)
        n140 = Bundle By Name(cluster=w202, "No. Channels"=w198, "Sample Rate"=w204, "Header size"=w203, "Data -> 3D Coil"=w197) -> (w200:T2)
        n141 = Bundle By Name(cluster=w229, "Selected Data File"=w201, "Rex Data File"=w200) -> (w230:T8)
        n142 = local write "Rex Data File"(w200) -> ()
      }
      frame "Sort 6 Field/Int Channels" {
        w999 = dbl[][] []
        n143 = Unbundle By Name(w1000) -> ("Coil 0 (Head) : Coil 1 (Left Eye) : Coil 2 (Right Eye)"=w1002:T4, "Addtional Channels"=w1001:T3, "Rex Data File.Data -> 3D Coil"=w990:dbl[][], "Field Gains"=w989:i32[][])
        n144 = for {
          tunnel: w1002 -> [w1045] mode=indexing
          shift-right: [w1035] -> w994
          shift-left: w999 -> [w1036]
          tunnel: w990 -> [w1034]
          n145 = Unbundle By Name(w1045) -> ("Dir and X field channel No."=w1028:i32, "Dir and Y field channel No."=w1029:i32, "Dir and Z field channel No."=w1030:i32, "Tor and X field channel No."=w1031:i32, "Tor and Y field channel No."=w1032:i32, "Tor and Z field channel No."=w1033:i32, "Common Offset Factor"=w1044:dbl, "Common Scaling Factor"=w1042:dbl)
          n146 = Subtract(x=w1034, y=w1044) -> (x-y=w1043:dbl[][])
          n147 = Multiply(x=w1043, y=w1042) -> (x*y=w1041:dbl[][])
          n148 = Index Array(array=w1041, index (row)=w1028) -> (element=w1040:dbl[])  [unwired: 1 in]
          n149 = Index Array(array=w1041, index (row)=w1029) -> (element=w1039:dbl[])  [unwired: 1 in]
          n150 = Index Array(array=w1041, index (row)=w1030) -> (element=w1038:dbl[])  [unwired: 1 in]
          n151 = Index Array(array=w1041, index (row)=w1031) -> (element=w1027:dbl[])  [unwired: 1 in]
          n152 = Index Array(array=w1041, index (row)=w1032) -> (element=w1026:dbl[])  [unwired: 1 in]
          n153 = Index Array(array=w1041, index (row)=w1033) -> (element=w1025:dbl[])  [unwired: 1 in]
          n154 = Build Array(w1040, w1039, w1038, w1027, w1026, w1025) -> (w1037:dbl[][])
          n155 = Build Array (concatenate)(w1036, w1037) -> (w1035:dbl[][])
        }
        n156 = for {
          tunnel: w1001 -> [w1024] mode=indexing
          tunnel: w990 -> [w1023]
          shift-right: [w1016] -> w991
          shift-left: w999 -> [w1017]
          n157 = Unbundle By Name(w1024) -> ("Channel No."=w1015:i32, "Offset Factor"=w1021:dbl, "Scaling Factor"=w1020:dbl)
          n158 = Index Array(array=w1023, index (row)=w1015) -> (element=w1022:dbl[])  [unwired: 1 in]
          n159 = Subtract(x=w1022, y=w1021) -> (x-y=w1019:dbl[])
          n160 = Multiply(x=w1019, y=w1020) -> (x*y=w1018:dbl[])
          n161 = Build Array (concatenate)(w1017, w1018) -> (w1016:dbl[][])
        }
        n162 = for {
          tunnel: w989 -> [w1012]
          tunnel: w989 -> [_] mode=indexing
          shift-right: [w1005] -> w992
          shift-left: i32[][] [] -> [w1006]
          i -> [w1014]
          n163 = Multiply(x=2, y=w1014) -> (x*y=w1011:i32)
          n164 = Increment(x=w1011) -> (x+1=w1010:i32)
          n165 = Index Array(array=w1012, index (col)=w1011) -> (element=w1009:i32[])  [unwired: 1 in]
          n166 = Index Array(array=w1012, index (col)=w1010) -> (element=w1008:i32[])  [unwired: 1 in]
          n167 = Build Array (concatenate)(w1009, w1008) -> (w1007:i32[])
          n168 = Build Array (concatenate)(w1007, w1006) -> (w1005:i32[][])
        }
        n169 = local read "Rex Data File"() -> (w996:T2)
        n170 = Bundle By Name(cluster=w996, "Data -> 3D Coil"=w994, "Data -> Additional"=w991) -> (w995:T2)
        n171 = Bundle By Name(cluster=w1000, "Field Gains"=w992, "Rex Data File"=w995) -> (w997:T8)
        n172 = local write "Rex Data File"(w995) -> ()
      }
      frame "Calculate 6 Field/Int Rot Matrix" {
        w1077 = dbl[][] []
        n173 = Unbundle By Name(w1075) -> ("Addtional Channels"=w1063:T3, "Rex Data File.Data -> Additional"=w1052:dbl[][], "Rex Data File.Sample Rate"=w1053:i32, "Rex Data File.Data -> 3D Coil"=w1062:dbl[][], "Channel Plot DY DZ for H LE RE"=w1081:i32[], "Coil 0 (Head) : Coil 1 (Left Eye) : Coil 2 (Right Eye)"=w1080:T4, "Field Gains"=w1079:i32[][])
        n174 = Build Array (concatenate)(w1062, w1052) -> (w1061:dbl[][])
        n175 = for {
          tunnel: w1081 -> [w1224] mode=indexing
          tunnel: w1061 -> [w1225]
          shift-right: [w1221] -> w1076
          shift-left: w1077 -> [w1223]
          n176 = Array Subset(array=w1225, index (row)=w1224, length (row)=1 ("Array Length"), index (col)=0 ("Array Index"), length (col)=15000 ("Array Length")) -> (w1222:dbl[][])
          n177 = Build Array (concatenate)(w1223, w1222) -> (w1221:dbl[][])
        }
        n178 = call "Select Reference.vi"("3D Coil"=w1076) -> ("References"=w1078:i32[])
        n179 = for {
          tunnel: w1080 -> [_] mode=indexing
          tunnel: w1062 -> [w1215]
          tunnel: w1079 -> [w1214]
          tunnel: w1078 -> [w1211] mode=indexing
          shift-right: [w1209] -> w1074
          shift-left: w1077 -> [w1208]
          tunnel: ["3D Convention"] -> w1073
          i -> [w1205]
          w1216 = 6 ("x")
          n180 = Multiply(x=w1205, y=w1216) -> (x*y=w1217:i32)
          n181 = Not Equal To 0?(x=w1205) -> (x != 0?=w1204:bool)
          n182 = Index Array(array=w1214, index (row)=w1205) -> (element=w1212:i32[])  [unwired: 1 in]
          n183 = Array Subset(array=w1215, index (row)=w1217, length (row)=w1216) -> (w1213:dbl[][])  [unwired: 2 in]
          n184 = And(x="LE and RE 2D coils", y=w1204) -> (x .and. y?=w1202:bool)
          n185 = call "3 D Ang Pos for 6 Field-Int.vi"("With Respect To:"=enum16{"Referenced", "UnReferenced"}."Referenced", "LE and RE 2D coils"=w1202, "Reference index"=w1211, "3D Convention"="3D Convention", "Field Gains"=w1212, "3D Voltage Data"=w1213) -> ("3D Position"=w1210:dbl[][])  [unwired: 5 in]
          n186 = Build Array (concatenate)(w1208, w1210) -> (w1209:dbl[][])
        }
        n187 = case shown="True" "Case Constant\n(See Context Help)" {
          tunnel: w1074 -> [w1105 w1116]
          tunnel: w1073 -> [w1104 w1115]
          tunnel: [w1103 w1108] -> w1072
          tunnel: [w1102 w1108] -> w1071
          tunnel: [w1101 w1108] -> w1070
          tunnel: [w1100 w1114] -> w1069
          tunnel: [w1099 w1113] -> w1068
          tunnel: [w1098 w1108] -> w1067
          tunnel: [w1097 w1109] -> w1060
          tunnel: [w1096 w1109] -> w1059
          tunnel: [w1095 w1109] -> w1058
          tunnel: [w1094 w1112] -> w1057
          tunnel: [w1093 w1111] -> w1056
          tunnel: [w1092 w1109] -> w1055
          tunnel: w1053 -> [w1091 w1110]
          frame False {
            n188 = call "Head Co-ordinates 2.vi"("3D Convention"=w1104, "3D Type and Co-ordinate System"=T7."Position in Space", "Array"=w1105) -> ("Channel List"=w1097:string[], "3D Output"=w1103:dbl[][])  [unwired: 3 in]
            n189 = call "Head Co-ordinates 2.vi"("3D Convention"=w1104, "3D Type and Co-ordinate System"=T7."Position in Head", "Array"=w1105) -> ("Channel List"=w1094:string[], "3D Output"=w1100:dbl[][])  [unwired: 3 in]
            n190 = call "Head Co-ordinates 2.vi"("3D Convention"=w1104, "3D Type and Co-ordinate System"=T7."Velocity in Space", "Sample Rate"=w1091, "Array"=w1103) -> ("Channel List"=w1096:string[], "3D Output"=w1102:dbl[][])  [unwired: 2 in]
            n191 = call "Head Co-ordinates 2.vi"("3D Convention"=w1104, "3D Type and Co-ordinate System"=T7."Velocity in Head", "Sample Rate"=w1091, "Array"=w1100) -> ("Channel List"=w1093:string[], "3D Output"=w1099:dbl[][])  [unwired: 2 in]
            n192 = call "Head Co-ordinates 2.vi"("3D Type and Co-ordinate System"=T7."Acceleration in Space", "Sample Rate"=w1091, "Array"=w1102) -> ("Channel List"=w1095:string[], "3D Output"=w1101:dbl[][])  [unwired: 3 in]
            n193 = call "Head Co-ordinates 2.vi"("3D Type and Co-ordinate System"=T7."Acceleration in Head", "Sample Rate"=w1091, "Array"=w1099) -> ("Channel List"=w1092:string[], "3D Output"=w1098:dbl[][])  [unwired: 3 in]
          }
          frame True {
            w1108 = dbl[][] [] ("3D Output")
            w1109 = string[] [] ("Channel List")
            n194 = call "Head Co-ordinates 2.vi"("3D Convention"=w1115, "3D Type and Co-ordinate System"=T7."Position in Head", "Array"=w1116) -> ("Channel List"=w1112:string[], "3D Output"=w1114:dbl[][])  [unwired: 3 in]
            n195 = call "Head Co-ordinates 2.vi"("3D Convention"=w1115, "3D Type and Co-ordinate System"=T7."Velocity in Head", "Sample Rate"=w1110, "Array"=w1114) -> ("Channel List"=w1111:string[], "3D Output"=w1113:dbl[][])  [unwired: 2 in]
          }
        }
        n196 = for {
          tunnel: w1063 -> [_] mode=indexing
          tunnel: w1053 -> [w1123]
          tunnel: w1052 -> [w1121] mode=indexing
          shift-right: [w1119] -> w1051
          shift-left: dbl[][] [] -> [w1120]
          shift-right: [w1118] -> w1050
          shift-left: string[] [] -> [w1117]
          i -> [w1122]
          n197 = case shown="7" w1122 {
            tunnel: [w1128 w1134 w1136 w1143 w1153 w1163 w1173 w1179 w1185 w1191 w1197] -> w1118
            tunnel: w1123 -> [_ _ _ w1151 w1161 w1171 _ _ _ _ _]
            tunnel: [w1127 w1133 w1139 w1150 w1160 w1170 w1175 w1181 w1187 w1193 w1199] -> w1119
            tunnel: w1121 -> [w1125 w1131 w1140 w1148 w1158 w1168 w1176 w1182 w1188 w1194 w1200]
            tunnel: w1120 -> [w1126 w1132 w1141 w1146 w1156 w1166 w1177 w1183 w1189 w1195 w1201]
            tunnel: w1117 -> [w1129 w1135 w1138 w1142 w1152 w1162 w1174 w1180 w1186 w1192 w1198]
            frame 0, Default {
              n198 = Build Array (concatenate)(w1126, w1125) -> (w1127:dbl[][])
              n199 = Build Array (concatenate)(w1129, "Chair Position") -> (w1128:string[])
            }
            frame 1 {
              n200 = Build Array (concatenate)(w1132, w1131) -> (w1133:dbl[][])
              n201 = Build Array (concatenate)(w1135, "Chair Velocity") -> (w1134:string[])
            }
            frame 2 {
              n202 = Build Array (concatenate)(w1138, "Button") -> (w1136:string[])
              n203 = Build Array (concatenate)(w1141, w1140) -> (w1139:dbl[][])
            }
            frame 3 {
              n204 = Build Array(w1148) -> (w1147:dbl[][])
              n205 = call "Differentiate 3D.vi"("Sample Rate 4"=w1151, "Data (in)"=w1147) -> ("Data (differentiated)"=w1149:dbl[][])  [unwired: 3 in]
              n206 = Build Array (concatenate)(w1142, "Ascension X or ch25", "Ascension X Vel") -> (w1143:string[])
              n207 = Build Array (concatenate)(w1146, w1147, w1149) -> (w1150:dbl[][])
            }
            frame 4 {
              n208 = Build Array(w1158) -> (w1157:dbl[][])
              n209 = call "Differentiate 3D.vi"("Sample Rate 4"=w1161, "Data (in)"=w1157) -> ("Data (differentiated)"=w1159:dbl[][])  [unwired: 3 in]
              n210 = Build Array (concatenate)(w1152, "Ascension Y", "Ascension Y Vel") -> (w1153:string[])
              n211 = Build Array (concatenate)(w1156, w1157, w1159) -> (w1160:dbl[][])
            }
            frame 5 {
              n212 = Build Array(w1168) -> (w1167:dbl[][])
              n213 = call "Differentiate 3D.vi"("Sample Rate 4"=w1171, "Data (in)"=w1167) -> ("Data (differentiated)"=w1169:dbl[][])  [unwired: 3 in]
              n214 = Build Array (concatenate)(w1162, "Ascension Z", "Ascension Z Vel") -> (w1163:string[])
              n215 = Build Array (concatenate)(w1166, w1167, w1169) -> (w1170:dbl[][])
            }
            frame 6 {
              n216 = Build Array (concatenate)(w1174, "Ascension q0") -> (w1173:string[])
              n217 = Build Array (concatenate)(w1177, w1176) -> (w1175:dbl[][])
            }
            frame 7 {
              n218 = Build Array (concatenate)(w1180, "Ascension q1") -> (w1179:string[])
              n219 = Build Array (concatenate)(w1183, w1182) -> (w1181:dbl[][])
            }
            frame 8 {
              n220 = Build Array (concatenate)(w1186, "Ascension q2") -> (w1185:string[])
              n221 = Build Array (concatenate)(w1189, w1188) -> (w1187:dbl[][])
            }
            frame 9 {
              n222 = Build Array (concatenate)(w1192, "Ascension q3") -> (w1191:string[])
              n223 = Build Array (concatenate)(w1195, w1194) -> (w1193:dbl[][])
            }
            frame 10 {
              n224 = Build Array (concatenate)(w1198, "LED") -> (w1197:string[])
              n225 = Build Array (concatenate)(w1201, w1200) -> (w1199:dbl[][])
            }
          }
        }
        n226 = Build Array (concatenate)(w1060, w1059, w1058, w1057, w1056, w1055, w1050, string[] [" "] ("Input Array")) -> (w1054:string[])
        n227 = Build Array (concatenate)(w1072, w1071, w1070, w1069, w1068, w1067, w1051) -> (w1066:dbl[][])
        n228 = Bundle By Name(cluster=w1075, "All Data.Data Channels"=w1066, "All Data.Sample Rate"=w1053, "All Data.Channel List"=w1054) -> (w1065:T8)
        n229 = Unbundle By Name(w1065) -> ("All Data"=→"All Data":T5)
      }
      frame "Export Channels" {
        n230 = Unbundle By Name(w1231) -> ("All Data.Sample Rate"=w1232:i32, "All Data.Data Channels"=w1230:dbl[][], "All Data.Channel List"=w1227:string[])
        n231 = property on="Ring" class="Ring (strict)"("Strings []"=w1227) -> ()  [unwired: 2 in, 2 out]
        n232 = for {
          tunnel: w1230 -> [w1242]
          tunnel: "Export Channel List" -> [w1239] mode=indexing
          tunnel: [w1241] -> w1228 mode=indexing
          tunnel: w1227 -> [w1240]
          tunnel: [w1238] -> w1226 mode=indexing
          n233 = Index Array(array=w1240, index=w1239) -> (element=w1238:string)
          n234 = Index Array(array=w1242, index (row)=w1239) -> (element=w1241:dbl[])  [unwired: 1 in]
        }
        n235 = local read "Data Export"() -> (w1234:T5)
        n236 = Bundle By Name(cluster=w1234, "Sample Rate"=w1232, "Data Channels"=w1228, "Channel List"=w1226) -> (→"Data Export":T5)
      }
      frame "Stop" {
      }
      frame "Quit", Default {
      }
    }
  }
